vi "Grow.vi"(8 "error in (no error)":errorcluster, 11 "Animal in":refnum<class "Animal.lvclass">) -> (0 "error out":errorcluster, 3 "Animal out":refnum<class "Animal.lvclass">)   [LabVIEW 2024, in "Animal.lvclass"]
doc: "本VI是为《我和LabVIEW》一书编写的示例。\n关于本书的介绍请参考网页：\nhttp://ruanqizhen.spaces.live.com/blog/cns!5852D4F797C53FB6!4310.entry"
uses:
  Animal.lvclass
  Animal.lvclass/Animal.ctl
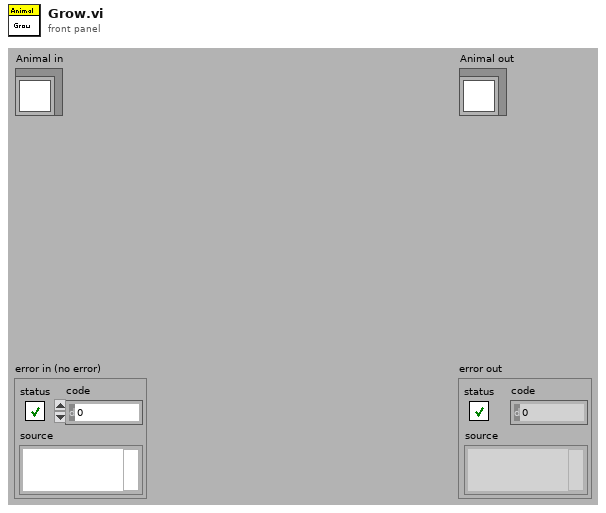
[diagram p1: front panel]
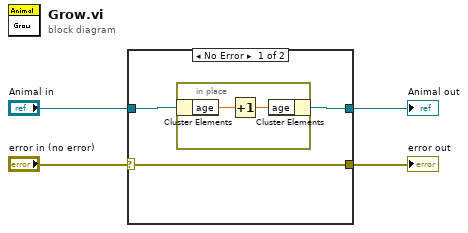
[diagram p0: block diagram]
diagram:
  n1 = case shown="No Error" "error in (no error)" {
    selector: "error in (no error)" -> [w7 w11]
    tunnel: [w7 w11] -> w3
    tunnel: [w5 w10] -> w1
    tunnel: "Animal in" -> [w6 w10]
    frame No Error {
      n2 = in-place {
        n3 = in-place-cluster #1(w6) -> ("age"=w9:dbl)
        n4 = Increment(x=w9) -> (x+1=w8:dbl)
        n5 = in-place-cluster #1("age"=w8) -> (w5:refnum<class "Animal.lvclass">)
      }
    }
    frame Error {
    }
  }
  "error out" <- w3
  "Animal out" <- w1
